vi "LIAbench.vi"() -> ()   [LabVIEW 2016]
uses:
  <vilib>/ErrorRing/Error Ring.xnode
  <instrlib>/Stanford Research SR865/Stanford Research SR865.lvlib
panel:
  in  "OK Button":bool
  in  "Response":string
  in  "Command":string
  out "LIA Connected":bool
  in  "Connect":bool
  in  "VISA adress":string
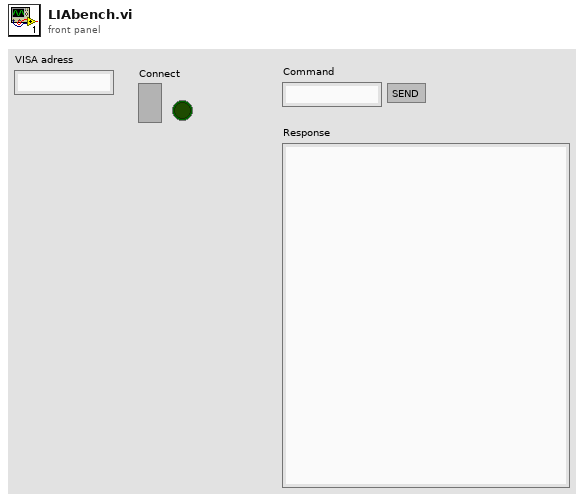
[diagram p1: front panel]
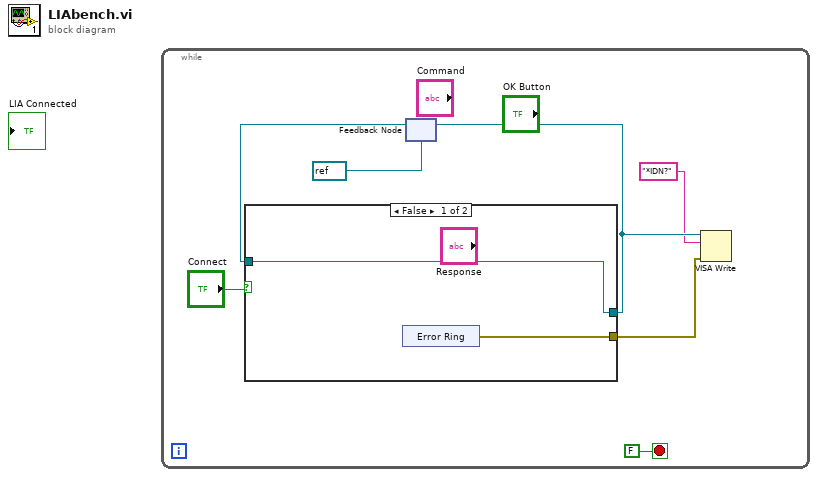
[diagram p0: block diagram]
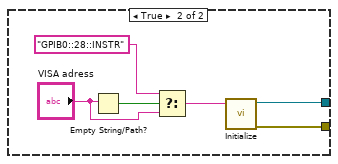
[diagram p2: hidden frame]
diagram:
  n1 = while {
    stop <- FALSE stop-if-true
    n2 = feedback #1(refnum<visa-resource-name> refnum ("VISA resource name out")) -> (w5:refnum<visa-resource-name>)
    n3 = case shown="False" "Connect" {
      tunnel: [w9 w12] -> w3
      tunnel: w5 -> [w9 _]
      tunnel: [w8 w11] -> w2
      frame False {
        n4 = xnode "Error Ring"() -> ("error out"=w8:errorcluster)
      }
      frame True {
        n5 = Empty String/Path?(string/path="VISA adress") -> (empty?=w13:bool)
        n6 = Select(t="GPIB0::28::INSTR", s=w13, f="VISA adress") -> (s? t:f=w16:string)
        n7 = call <instrlib>:"Initialize.vi"("VISA resource name"=w16) -> ("error out"=w11:errorcluster, "VISA resource name out"=w12:refnum<visa-resource-name>)  [unwired: 9 in]
      }
    }
    n8 = feedback-in #1(w3) -> ()
    n9 = VISA Write(VISA resource name=w3, write buffer="*IDN?", error in (no error)=w2) -> ()  [unwired: 3 out]
  }
